vi "discover channels.vi"(8 "error in":errorcluster, 10 "module configuration":refnum<class "TBM module configuration.lvclass">, 11 "module in":refnum<class "TBM module execution interface.lvclass">) -> (0 "error out":errorcluster, 2 "updated configuration":refnum<class "TBM module configuration.lvclass">, 3 "module out":refnum<class "TBM module execution interface.lvclass">)   [LabVIEW 2013, in "TBM module execution interface.lvclass"]
doc: "Provides an interface for discovering channels at runtime. While this interface performs no operations, a child should provide an override which performs discovery of any channel information that may be available at run time and not at configure time."
uses:
  TBM module execution interface.lvclass
  module configuration/TBM module configuration.lvclass
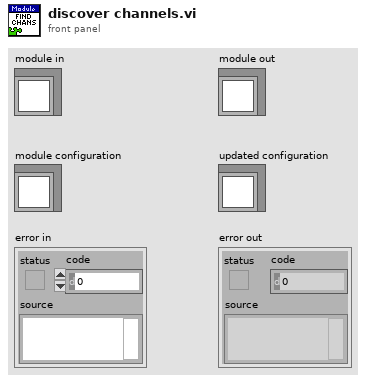
[diagram p1: front panel]
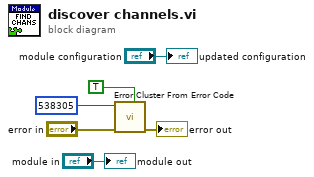
[diagram p0: block diagram]
diagram:
  n1 = call <vilib>:"Error Cluster From Error Code.vi"("is warning? (False)"=TRUE ("show call chain? (False)"), "error in (no error)"="error in", "error code (0)"=538305) -> ("error out"=→"error out":errorcluster)  [unwired: 6 in]
  "module out" <- "module in"
  "updated configuration" <- "module configuration"
